vi "Get Summary.vi"(8 "error in (no error)":errorcluster, 11 "Readiness Report":refnum<class "Readiness Report.lvclass">) -> (0 "error out":errorcluster, 3 "Summary":string)   [LabVIEW 2026, in "Readiness Report.lvclass"]
uses:
  Readiness Report.lvclass
  Readiness Report.lvclass/Readiness Report.ctl
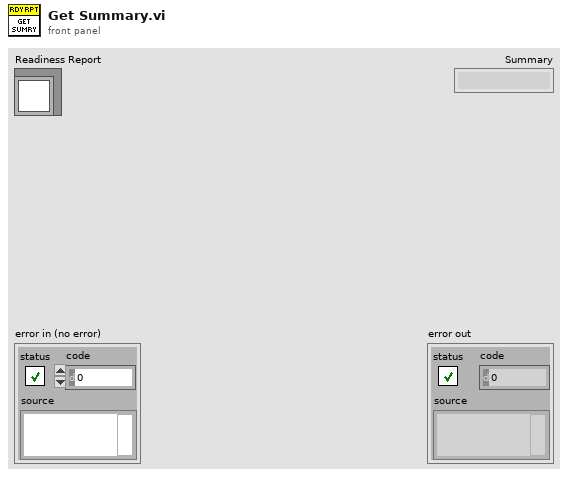
[diagram p1: front panel]
types:
  T1 = typedef "Readiness Check Result.ctl" = cluster{"Check Name":string, "State":T2, "Message":string}
  T2 = typedef "Readiness State Enum.ctl" = enum16{"Unknown", "Ready", "Warning", "NotReady"}
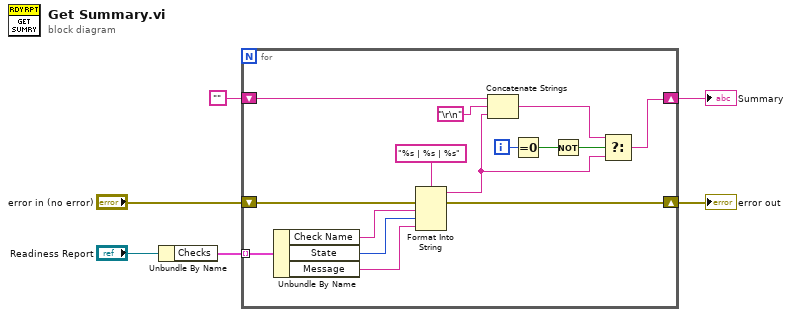
[diagram p0: block diagram]
diagram:
  n1 = Unbundle By Name("Readiness Report") -> ("Checks"=w5:T1[])
  n2 = for {
    tunnel: w5 -> [w21] mode=indexing
    shift-right: [w16] -> w2
    shift-left: "error in (no error)" -> [w7]
    shift-right: [w13] -> w1
    shift-left: "" -> [w11]
    i -> [w15]
    n3 = Unbundle By Name(w21) -> ("Check Name"=w19:string, "State"=w18:T2, "Message"=w17:string)
    n4 = Format Into String(format string="%s | %s | %s", error in=w7, w19, w18, w17) -> (resulting string=w9:string, error out=w16:errorcluster)  [unwired: 1 in]
    n5 = Concatenate Strings(w11, "\r\n", w9) -> (w8:string)
    n6 = Equal To 0?(x=w15) -> (x = 0?=w14:bool)
    n7 = Not(x=w14) -> (.not. x?=w10:bool)
    n8 = Select(t=w8, s=w10, f=w9) -> (s? t:f=w13:string)
  }
  "error out" <- w2
  "Summary" <- w1
